vi "Write Starting Month.vi"(10 "Starting Month":u32) -> (3 "People By Month Wrapper out":refnum<class "People By Month Wrapper.lvclass">)   [LabVIEW 2023, in "People By Month Wrapper.lvclass"]
uses:
  People By Month Wrapper.lvclass
  People By Month Wrapper.lvclass/People By Month Wrapper.ctl
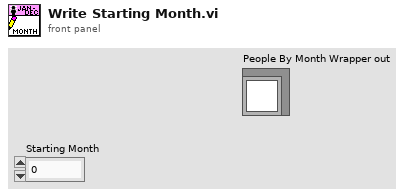
[diagram p1: front panel]
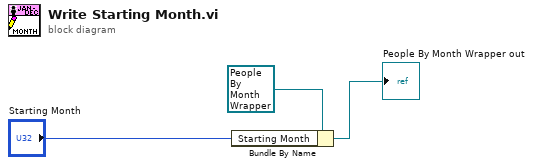
[diagram p0: block diagram]
diagram:
  n1 = Bundle By Name(cluster=refnum<class "People By Month Wrapper.lvclass"> refnum ("People By Month Wrapper in"), "Starting Month"="Starting Month") -> (→"People By Month Wrapper out":refnum<class "People By Month Wrapper.lvclass">)
